vi "cmc_chamber conditions.vi"() -> ()   [LabVIEW 2010]
panel:
  in  "stop":bool
  out "Chamber Condtions":T1 {"Pressure(mbar)" scale=600.0..1100.0; "Relative Humidity" scale=0.0..100.0 scale format="%#_3g"; "Temperature (Celsius)" scale=20.0..30.0}
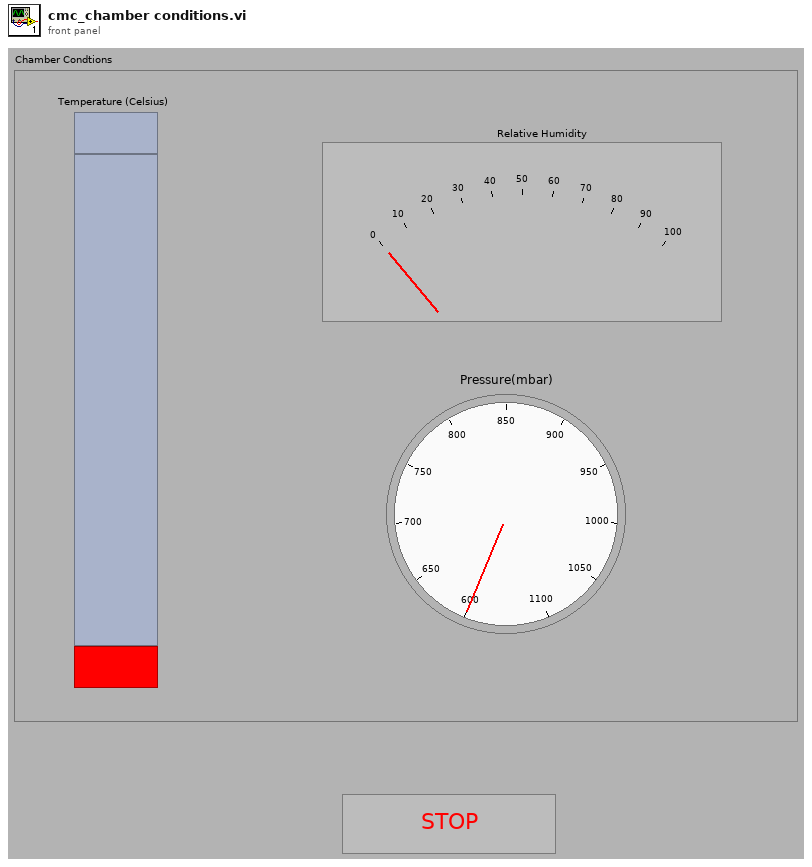
[diagram p1: front panel]
types:
  T1 = cluster{"Temperature (Celsius)":dbl, "Relative Humidity":dbl, "Pressure(mbar)":dbl}
  T2 = cluster{"Temp.":dbl, "Humidity":dbl, "Pressure":dbl}
  T3 = cluster{"T Voltage":dbl, "RH Voltage":dbl, "P Voltage":dbl}
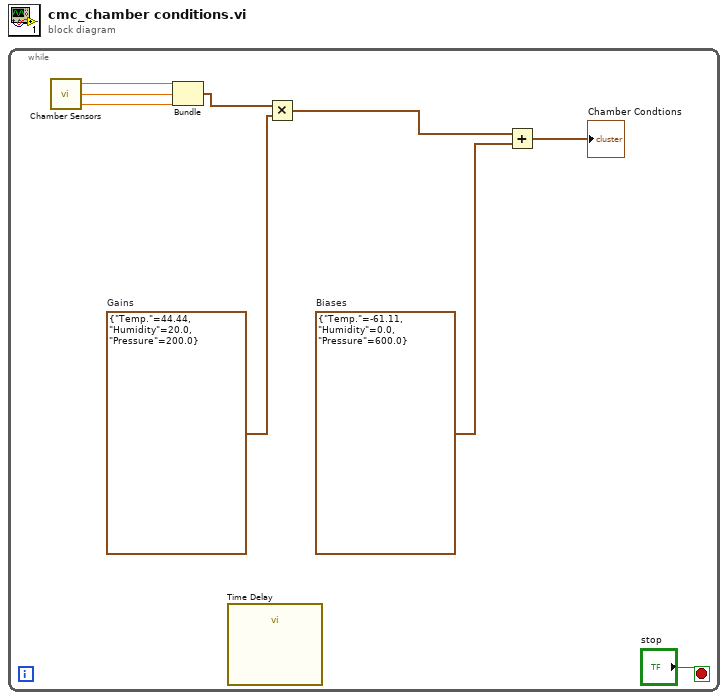
[diagram p0: block diagram]
diagram:
  n1 = while {
    stop <- "stop" stop-if-true
    w4 = T2 {"Temp."=-61.11, "Humidity"=0.0, "Pressure"=600.0}  # Biases
    w2 = T2 {"Temp."=44.44, "Humidity"=20.0, "Pressure"=200.0}  # Gains
    n2 = call "Chamber Sensors.vi"() -> ("P Voltage"=w7:dbl, "RH Voltage"=w8:dbl, "T Voltage"=w9:dbl)  [unwired: 3 in]
    n3 = Bundle("T Voltage"=w9, "RH Voltage"=w8, "P Voltage"=w7) -> (w6:T3)  [unwired: 1 in]
    n4 = call "Time Delay"() -> ()  [unwired: 11 in, 1 out]
    n5 = Multiply(x=w6, y=w2) -> (x*y=w5:cluster{dbl, dbl, dbl})
    n6 = Add(x=w5, y=w4) -> (x+y=→"Chamber Condtions":cluster{dbl, dbl, dbl})
  }
